vi "draw.a.vi"(11 "midi-ui in":refnum<class "midi-ui.lvclass">) -> (2 "coordinates":cluster{"x":dbl, "y":dbl}[](array[cluster]), 3 "midi-ui out":refnum<class "midi-ui.lvclass">)   [LabVIEW 2020, in "midi-ui.lvclass"]
uses:
  midi-ui.lvclass
  midi-ui.lvclass/midi-ui.ctl
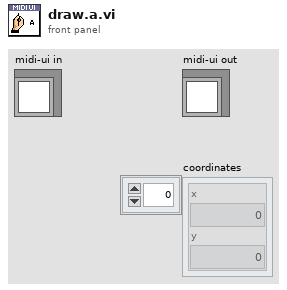
[diagram p1: front panel]
types:
  T1 = typedef "midi-ui.lvclass/privatedata.ctl" = cluster{"White Key Length":dbl, "White Key Width":dbl, "Black Key Length":dbl, "Polygon Corners by Name":map{string, cluster{"x":dbl, "y":dbl}[]}, "Anticlockwise rotations [0-3] (0)":i32, "Polygon Corners by Note Name":map{string, cluster{"x":dbl, "y":dbl}[]}, "Picture Control":refnum<vi>, "Owning VI":refnum<vi>, "Control Index":i32, "Note Bounds by Note Name":map{string, cluster{"max":dbl, "min":dbl}}, "Notes on screen":cluster{"Note Value":enum8{"C-2", "C#-2", "D-2", "D#-2", "E-2", "F-2", "F#-2", "G-2", "G#-2", "A-2", "A#-2", "B-2", "C-1", "C#-1", "D-1", "D#-1", "E-1", "F-1", "F#-1", "G-1", "G#-1", "A-1", "A#-1", "B-1", "C0", "C#0", "D0", "D#0", "E0", "F0", "F#0", "G0", "G#0", "A0", "A#0", "B0", "C1", "C#1", "D1", "D#1", "E1", "F1", "F#1", "G1", "G#1", "A1", "A#1", "B1", "C2", "C#2", "D2", "D#2", "E2", "F2", "F#2", "G2", "G#2", "A2", "A#2", "B2", "C3", "C#3", "D3", "D#3", "E3", "F3", "F#3", "G3", "G#3", "A3", "A#3", "B3", "C4", "C#4", "D4", "D#4", "E4", "F4", "F#4", "G4", "G#4", "A4", "A#4", "B4", "C5", "C#5", "D5", "D#5", "E5", "F5", "F#5", "G5", "G#5", "A5", "A#5", "B5", "C6", "C#6", "D6", "D#6", "E6", "F6", "F#6", "G6", "G#6", "A6", "A#6", "B6", "C7", "C#7", "D7", "D#7", "E7", "F7", "F#7", "G7", "G#7", "A7", "A#7", "B7", "C8", "C#8", "D8", "D#8", "E8", "F8", "F#8", "G"}, "End Time":u32, "Start Time":u32}[], "Polygon Pictures by Note Name":map{i32, cluster{"Note On":picture, "Note Off":picture}}, "keyboard":picture[], "Keyboard Note Index by Name":map{i32, i32}, "music":picture[]}
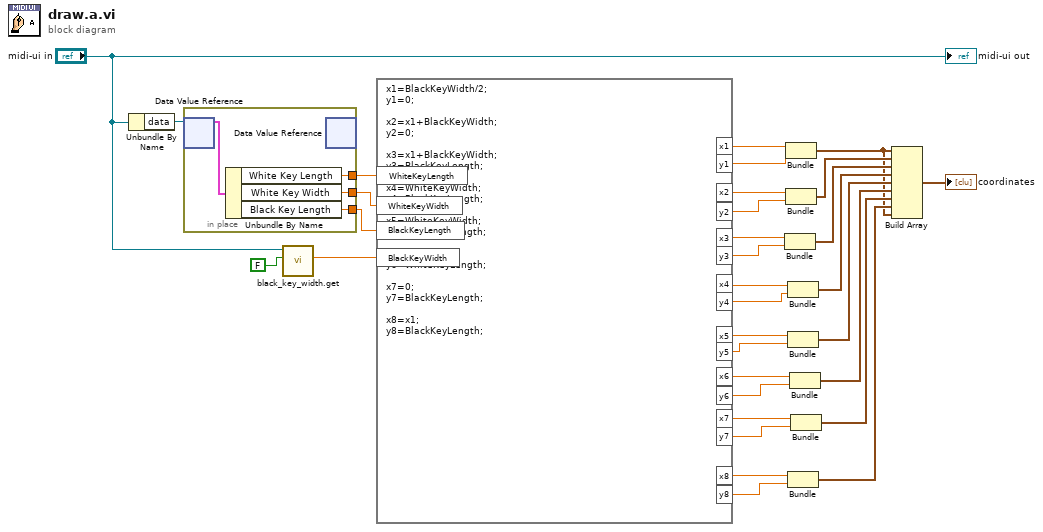
[diagram p0: block diagram]
diagram:
  n1 = Unbundle By Name("midi-ui in") -> ("data"=w5:refnum<data-value>)
  n2 = in-place {
    in-place-border: [w35] -> w3
    in-place-border: [w34] -> w2
    in-place-border: [w33] -> w1
    n3 = in-place-dvr #1(w5) -> (w36:T1)  [unwired: 1 out]
    n4 = Unbundle By Name(w36) -> ("White Key Length"=w35:dbl, "White Key Width"=w34:dbl, "Black Key Length"=w33:dbl)
    n5 = in-place-dvr #1() -> ()  [unwired: 1 in, 2 out]
  }
  n6 = call "black_key_width.get.vi"("C# or D#?"=FALSE, "midi-ui in"="midi-ui in") -> ("Black Key Width"=w7:dbl)  [unwired: 8 in, 1 out]
  n7 = formula code="x1=BlackKeyWidth/2;\ny1=0;\n\nx2=x1+BlackKeyWidth;\ny2=0;\n\nx3=x1+BlackKeyWidth;\ny3=BlackKeyLength;\n\nx4=WhiteKeyWidth;\ny4=BlackKeyLength;\n\nx5=WhiteKeyWidth;\ny5=WhiteKeyLength;\n\nx6=0;\ny6=WhiteKeyLength;\n\nx7=0;\ny7=BlackKeyLength;\n\nx8=x1;\ny8=BlackKeyLength;"("WhiteKeyLength"=w3, "WhiteKeyWidth"=w2, "BlackKeyLength"=w1, "BlackKeyWidth"=w7) -> ("x1"=w32:dbl, "y1"=w31:dbl, "x2"=w19:dbl, "y2"=w20:dbl, "x3"=w21:dbl, "y3"=w30:dbl, "x4"=w22:dbl, "y4"=w23:dbl, "x6"=w24:dbl, "y6"=w25:dbl, "x7"=w26:dbl, "y7"=w27:dbl, "x8"=w28:dbl, "y8"=w29:dbl, "x5"=w11:dbl, "y5"=w12:dbl)
  n8 = Bundle("x3"=w21, "y3"=w30) -> (w17:cluster{"x3":dbl, "y3":dbl})  [unwired: 1 in]
  n9 = Bundle("x1"=w32, "y1"=w31) -> (w9:cluster{"x1":dbl, "y1":dbl})  [unwired: 1 in]
  n10 = Bundle("x2"=w19, "y2"=w20) -> (w18:cluster{"x2":dbl, "y2":dbl})  [unwired: 1 in]
  n11 = Bundle("x4"=w22, "y4"=w23) -> (w16:cluster{"x4":dbl, "y4":dbl})  [unwired: 1 in]
  n12 = Bundle("x5"=w11, "y5"=w12) -> (w10:cluster{"x5":dbl, "y5":dbl})  [unwired: 1 in]
  n13 = Bundle("x8"=w28, "y8"=w29) -> (w13:cluster{"x8":dbl, "y8":dbl})  [unwired: 1 in]
  n14 = Bundle("x6"=w24, "y6"=w25) -> (w15:cluster{"x6":dbl, "y6":dbl})  [unwired: 1 in]
  n15 = Bundle("x7"=w26, "y7"=w27) -> (w14:cluster{"x7":dbl, "y7":dbl})  [unwired: 1 in]
  n16 = Build Array(w9, w18, w17, w16, w10, w15, w14, w13, w9) -> (→"coordinates":cluster{"x1":dbl, "y1":dbl}[])
  "midi-ui out" <- "midi-ui in"
